vi "MM Multi DOF Status DAO.vi"(8 "error in (no error)":errorcluster, 10 "Mixed Mode Multidof Status In":T1, 11 "Actions":T4) -> (0 "error out":errorcluster, 2 "Mixed Mode Multidof Status Out":T1)   [LabVIEW 2013]
uses:
  Data Access Objects/Metadata/DAO Actions.ctl
  Mixed Mode Multidof Status.ctl
  Mixed Mode Multidof State.ctl
  Apps/Yes No Button.ctl
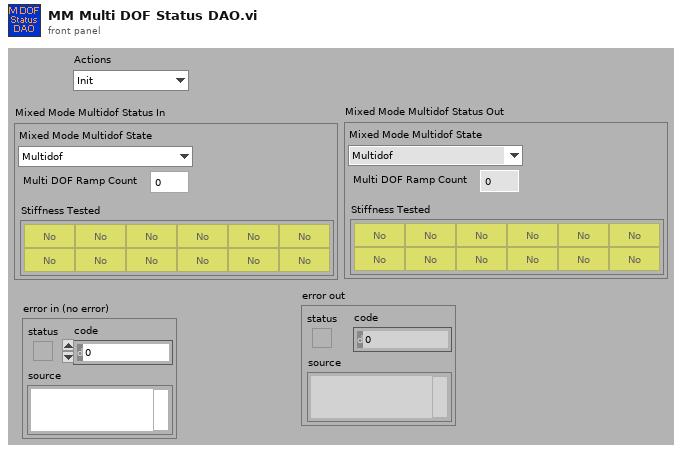
[diagram p1: front panel]
types:
  T1 = typedef "Mixed Mode Multidof Status.ctl" = cluster{"Mixed Mode Multidof State":T2, "Multi DOF Ramp Count":i32, "Stiffness Tested":T3[][]}
  T2 = typedef "Mixed Mode Multidof State.ctl" = enum16{"Multidof", "Stiffness Test", "Start Iterative Stage"}
  T3 = typedef "Yes No Button.ctl" = bool
  T4 = typedef "DAO Actions.ctl" = enum16{"Init", "Get", "Set"}
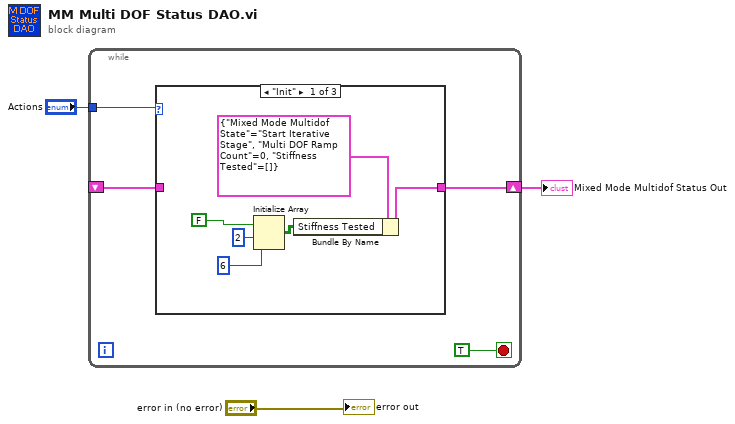
[diagram p0: block diagram]
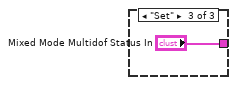
[diagram p3: hidden frame]
diagram:
  n1 = while {
    tunnel: "Actions" -> [w6]
    shift-right: [w5] -> w1
    shift-left: _ -> [w4]
    stop <- TRUE stop-if-true
    n2 = case shown="\"Init\"" w6 {
      tunnel: [w12 w14 "Mixed Mode Multidof Status In"] -> w5
      tunnel: w4 -> [_ w14 _]
      frame "Init" {
        n3 = Initialize Array(FALSE, 2 ("dimension size"), 6 ("dimension size")) -> (w8:bool[][])
        n4 = Bundle By Name(cluster=T1 {"Mixed Mode Multidof State"=enum."Start Iterative Stage", "Multi DOF Ramp Count"=0, "Stiffness Tested"=[]} ("Mixed Mode Multidof Status In"), "Stiffness Tested"=w8) -> (w12:T1)
      }
      frame "Get" {
      }
      frame "Set" {
      }
    }
  }
  "Mixed Mode Multidof Status Out" <- w1
  "error out" <- "error in (no error)"
